vi "[Benchmark] RT Loop - System Health and FPGA Monitoring.vi"(8 "error in (no error)":errorcluster, 9 "FPGA VI Reference":T1, 10 "Session in":refnum<k21>, 11 "Message Queue":refnum<queue>) -> (3 "Session out":refnum<k21>)   [LabVIEW 2017]
uses:
  UI Error Handlers/support/Message Queue/Message Cluster.ctl
  controls/FPGA VI Reference.ctl
  controls/CPU Loads.ctl
  controls/FPGA State.ctl
  <vilib>/Utility/error.llb/Error Cluster From Error Code.vi
  <vilib>/rvi/errors/niLvFpgaAdjustHostInterfaceError.vi
  <vilib>/rvi/interface/nirviReadWriteControl/nirviReadWriteControl.xnode
  <vilib>/NI_Real-Time Target Support.lvlib
  <resource>/objmgr/nisysapi.rc
  NiFpgaLv.dll
  <vilib>/rvi/interface/Simulation/niFpgaSimulationCallBeginRW.vi
  UI Error Handlers/support/Message Queue/Message Queue.lvlib
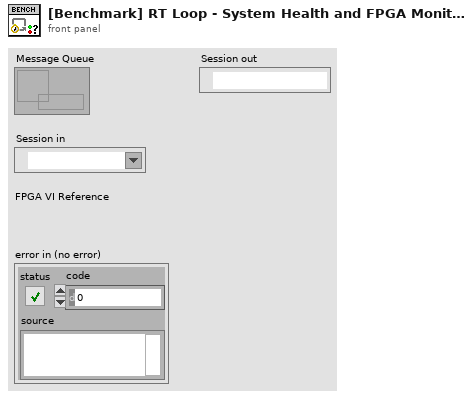
[diagram p1: front panel]
types:
  T1 = typedef "FPGA VI Reference.ctl" = refnum<k20>
  T2 = typedef "NI_Real-Time Target Support.lvlib/RT CPU Load.ctl" = cluster{"Total (%)":dbl, "Time Critical (%)":dbl, "Timed Structures (%)":dbl, "High (%)":dbl, "Above Normal (%)":dbl, "Normal (%)":dbl, "Background (%)":dbl, "Idle (%)":dbl, "ISR (%)":dbl}
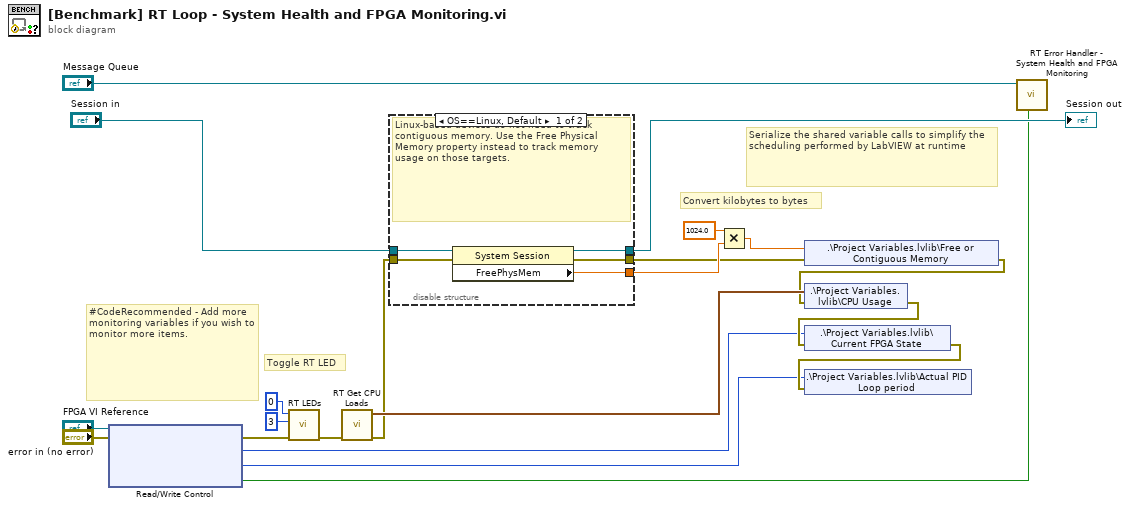
[diagram p0: block diagram]
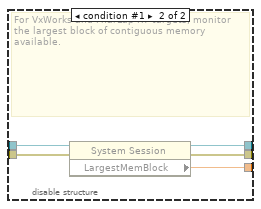
[diagram p2: hidden frame]
diagram:
  # "Convert kilobytes to bytes"
  # "Toggle RT LED"
  # "Serialize the shared variable calls to simplify the scheduling performed by LabVIEW at runtime"
  # "#CodeRecommended - Add more monitoring variables if you wish to monitor more items."
  n1 = xnode "Read/Write Control"("FPGA VI Reference In"="FPGA VI Reference", "error in"="error in (no error)") -> ("error out"=w13:errorcluster, "Current FPGA State"=w2:enum16{"Safe State", "Control (PID)"}, "PID Loop Period (tick)"=w1:u32, "Input Error"=w5:bool)  [unwired: 1 out]
  n2 = call <vilib>:"RT LEDs.vi"("error in (no error)"=w13, "State"=3, "LED Num"=0) -> ("error out"=w14:errorcluster)  [unwired: 3 in, 1 out]
  n3 = call <vilib>:"RT Get CPU Loads.vi"("error in (no error)"=w14) -> ("error out"=w17:errorcluster, "CPU loads"=w21:T2[])  [unwired: 9 in]
  n4 = disable-structure shown="OS==Linux, Default" {
    disable-tunnel: "Session in" -> [w26 w31]
    disable-tunnel: w17 -> [w25 w30]
    disable-tunnel: [w24 w29] -> w18
    disable-tunnel: [w23 w28] -> w19
    disable-tunnel: [w22 w27] -> w20
    frame condition #0 (active) {
      # "Linux-based devices do not need to track contiguous memory. Use the Free Physical Memory property instead to track memory usage on those targets."
      n5 = property class="System Session"(reference=w26, error in=w25) -> (reference out=w24:refnum<k21>, error out=w23:errorcluster, "FreePhysMem"=w22:dbl)
    }
    frame condition #1 {
      # "For VxWorks and PharLap RT targets, monitor the largest block of contiguous memory available."
      n6 = property class="System Session"(reference=w31, error in=w30) -> (reference out=w29:refnum<k21>, error out=w28:errorcluster, "LargestMemBlock"=w27:dbl)
    }
  }
  "Session out" <- w18
  n7 = Multiply(x=1024.0, y=w20) -> (x*y=w10:dbl)
  n8 = shared-variable ".\\Project Variables.lvlib\\Free or Contiguous Memory"(w10, error in=w19) -> (error out=w7:errorcluster)
  n9 = shared-variable ".\\Project Variables.lvlib\\CPU Usage"(w21, error in=w7) -> (error out=w8:errorcluster)
  n10 = shared-variable ".\\Project Variables.lvlib\\Current FPGA State"(w2, error in=w8) -> (error out=w6:errorcluster)
  n11 = shared-variable ".\\Project Variables.lvlib\\Actual PID Loop period"(w1, error in=w6) -> ()  [unwired: 1 out]
  n12 = call "RT Error Handler - System Health and FPGA Monitoring.vi"("Input Error (FPGA)"=w5, "Message Queue"="Message Queue") -> ()  [unwired: 9 in, 1 out]
